vi "SMR_LabVIEW_V1.vi"() -> ()   [LabVIEW 2025]
uses:
  <vilib>/DAQmx/read.llb/DAQmx Read (Analog 1D DBL NChan 1Samp).vi
  <vilib>/Analysis/baseanly.llb/Mean (DBL).vi
  <vilib>/DAQmx/create/channels.llb/DAQmx Create Channel (AI-Temperature-Thermocouple).vi
  <vilib>/DAQmx/create/channels.llb/DAQmx Create Channel (AI-Voltage-Basic).vi
  <vilib>/DAQmx/miscellaneous.llb/DAQmx Fill In Error Info.vi
  <vilib>/Analysis/NI_AALBase.lvlib
panel:
  out "Temperatures T1-T8 (deg C)":dbl[](array[numeric])
  out "Flow History":dbl(graph)
  out "Pressure History":dbl[](graph)
  out "Temperature History":dbl[](graph)
  out "Max Loop Pressure (psi)":dbl
  out "Average Loop Temp (deg C)":dbl
  out "Max Loop Temp (deg C)":dbl
  out "Heat Exchanger Flow (GPM)":dbl
  out "Raw NI9201 Voltages (V)":dbl[](array[numeric])
  out "Pressures P1-P7 (psi)":dbl[](array[numeric])
  in  "Loop Period (ms)":dbl=1000.0
  in  "Stop":bool
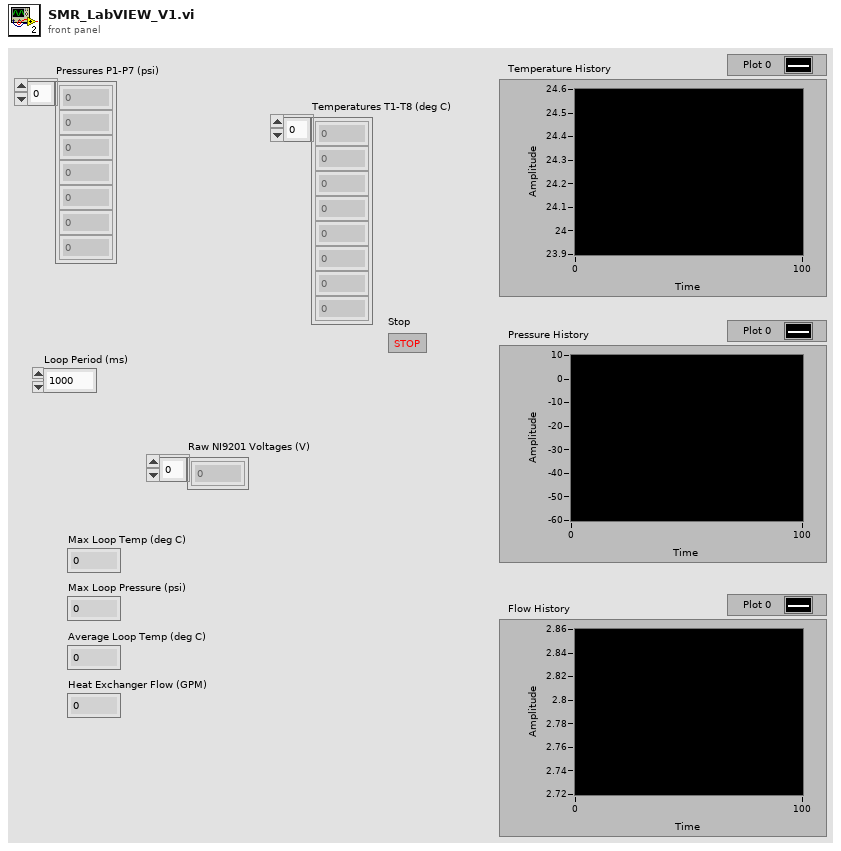
[diagram p1: front panel]
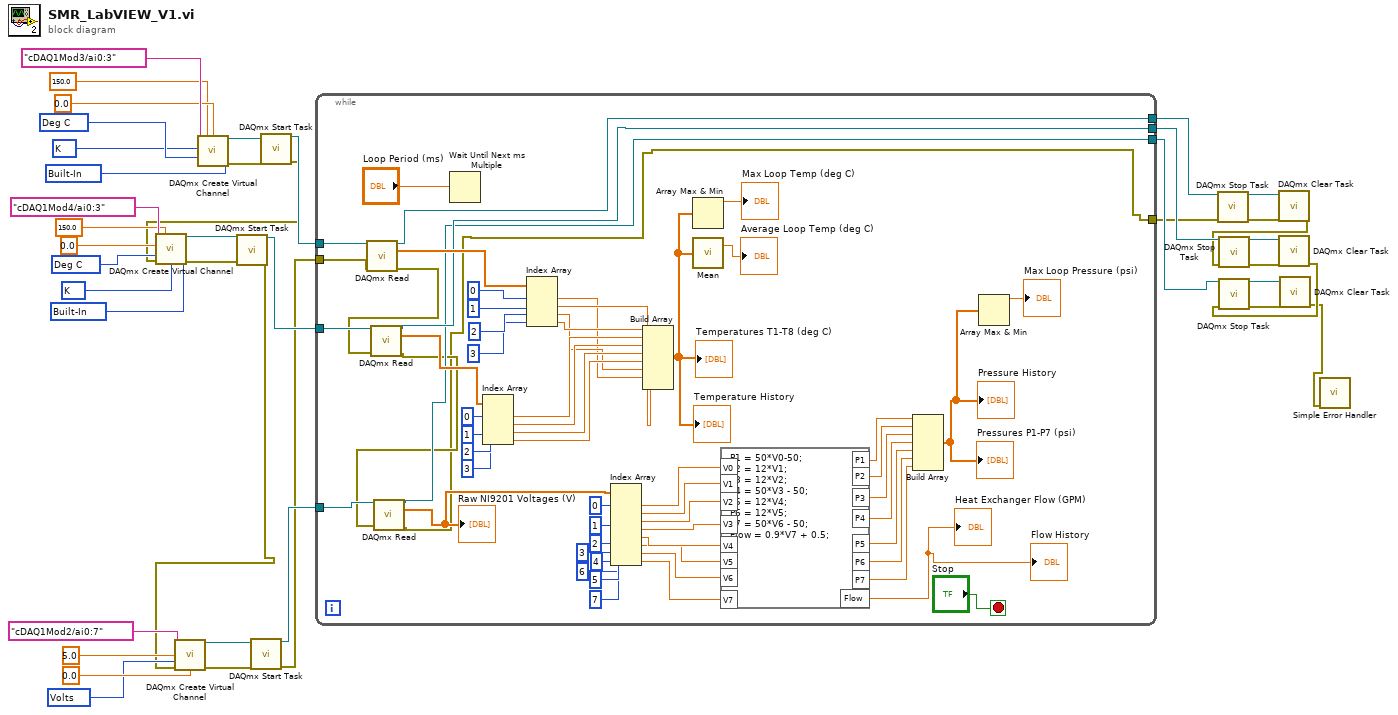
[diagram p0: block diagram]
diagram:
  w23 = 10348 items=["Volts"=10348, "From Custom Scale"=10065] ("units")
  w27 = 10200 items=["Built-In"=10200, "Constant Value"=10116, "Channel"=10113] ("cjc source")
  w28 = 10073 items=["J"=10072, "K"=10073, "N"=10077, "R"=10082, "S"=10085, "T"=10086, "B"=10047, "E"=10055] ("thermocouple type")
  w11 = 10143 items=["Deg C"=10143, "Deg F"=10144, "Kelvins"=10325, "Deg R"=10145, "From Custom Scale"=10065] ("units")
  w31 = 10200 items=["Built-In"=10200, "Constant Value"=10116, "Channel"=10113] ("cjc source")
  w32 = 10073 items=["J"=10072, "K"=10073, "N"=10077, "R"=10082, "S"=10085, "T"=10086, "B"=10047, "E"=10055] ("thermocouple type")
  w35 = 10143 items=["Deg C"=10143, "Deg F"=10144, "Kelvins"=10325, "Deg R"=10145, "From Custom Scale"=10065] ("units")
  n1 = call-poly <vilib>:"DAQmx Create Virtual Channel.vi"("maximum value"=150.0, "minimum value"=0.0, "physical channels"=tag "cDAQ1Mod3/ai0:3", "cjc source"=w31, "units"=w35, "thermocouple type"=w32) -> ("task out"=w40:refnum<k21>, "error out"=w39:errorcluster)  [unwired: 8 in]
  n2 = call <vilib>:"DAQmx Start Task.vi"("task/channels in"=w40, "error in"=w39) -> ("task out"=w20:refnum<k21>, "error out"=w10:errorcluster)  [unwired: 12 in]
  n3 = call-poly <vilib>:"DAQmx Create Virtual Channel.vi"("maximum value"=150.0, "minimum value"=0.0, "physical channels"=tag "cDAQ1Mod4/ai0:3", "cjc source"=w27, "units"=w11, "error in"=w10, "thermocouple type"=w28) -> ("task out"=w37:refnum<k21>, "error out"=w36:errorcluster)  [unwired: 7 in]
  n4 = call <vilib>:"DAQmx Start Task.vi"("task/channels in"=w37, "error in"=w36) -> ("task out"=w19:refnum<k21>, "error out"=w9:errorcluster)  [unwired: 12 in]
  n5 = call-poly <vilib>:"DAQmx Create Virtual Channel.vi"("maximum value"=5.0, "minimum value"=0.0, "physical channels"=tag "cDAQ1Mod2/ai0:7", "units"=w23, "error in"=w9) -> ("task out"=w22:refnum<k21>, "error out"=w21:errorcluster)  [unwired: 9 in]
  n6 = call <vilib>:"DAQmx Start Task.vi"("task/channels in"=w22, "error in"=w21) -> ("task out"=w18:refnum<k21>, "error out"=w8:errorcluster)  [unwired: 12 in]
  n7 = while {
    tunnel: w20 -> [w99]
    tunnel: w19 -> [w98]
    tunnel: w18 -> [w76]
    tunnel: [w48] -> w17
    tunnel: [w47] -> w16
    tunnel: [w46] -> w15
    tunnel: w8 -> [w45]
    tunnel: [w42] -> w7
    stop <- "Stop" stop-if-true
    n8 = call-poly <vilib>:"DAQmx Read.vi"("task/channels in"=w99, "error in"=w45) -> ("task out"=w48:refnum<k21>, "data"=w81:dbl[], "error out"=w44:errorcluster)  [unwired: 11 in]
    n9 = call-poly <vilib>:"DAQmx Read.vi"("task/channels in"=w98, "error in"=w44) -> ("task out"=w47:refnum<k21>, "data"=w80:dbl[], "error out"=w43:errorcluster)  [unwired: 11 in]
    n10 = call-poly <vilib>:"DAQmx Read.vi"("task/channels in"=w76, "error in"=w43) -> ("task out"=w46:refnum<k21>, "data"=w67:dbl[], "error out"=w42:errorcluster)  [unwired: 11 in]
    "Raw NI9201 Voltages (V)" <- w67
    n11 = Wait Until Next ms Multiple(millisecond multiple="Loop Period (ms)") -> ()  [unwired: 1 out]
    n12 = Index Array(array=w80, index #1=0 ("index"), index #2=1 ("index"), index #3=2 ("index"), index #4=3 ("index")) -> (element #1=w89:dbl, element #2=w88:dbl, element #3=w87:dbl, element #4=w86:dbl)
    n13 = Index Array(array=w81, index #1=0 ("index"), index #2=1 ("index"), index #3=2 ("index"), index #4=3 ("index")) -> (element #1=w82:dbl, element #2=w83:dbl, element #3=w84:dbl, element #4=w85:dbl)
    n14 = Index Array(array=w67, index #1=0 ("index"), index #2=1 ("index"), index #3=2 ("index"), index #4=3 ("index"), index #5=4 ("index"), index #6=5 ("index"), index #7=6 ("index"), index #8=7 ("index")) -> (element #1=w66:dbl, element #2=w65:dbl, element #3=w64:dbl, element #4=w63:dbl, element #5=w62:dbl, element #6=w61:dbl, element #7=w60:dbl, element #8=w59:dbl)
    n15 = Build Array(w85, w89, w88, w87, w86, w84, w82, w83) -> (w78:dbl[])
    "Temperatures T1-T8 (deg C)" <- w78
    "Temperature History" <- w78
    n16 = Array Max & Min(array=w78) -> (max value=→"Max Loop Temp (deg C)":dbl)  [unwired: 3 out]
    n17 = call-poly <vilib>:"Mean.vi"("X"=w78) -> ("mean"=→"Average Loop Temp (deg C)":dbl)  [unwired: 1 out]
    n18 = formula code="P1 = 50*V0-50;\nP2 = 12*V1;\nP3 = 12*V2;\nP4 = 50*V3 - 50;\nP5 = 12*V4;\nP6 = 12*V5; \nP7 = 50*V6 - 50;\nFlow = 0.9*V7 + 0.5;"("V0"=w66, "V1"=w65, "V2"=w64, "V3"=w63, "V4"=w62, "V5"=w61, "V6"=w60, "V7"=w59) -> ("P1"=w58:dbl, "P2"=w57:dbl, "P3"=w56:dbl, "P4"=w55:dbl, "P5"=w54:dbl, "P6"=w53:dbl, "P7"=w52:dbl, "Flow"=→"Heat Exchanger Flow (GPM)" →"Flow History":dbl)
    n19 = Build Array(w58, w57, w56, w55, w54, w53, w52) -> (w51:dbl[])
    "Pressures P1-P7 (psi)" <- w51
    "Pressure History" <- w51
    n20 = Array Max & Min(array=w51) -> (max value=→"Max Loop Pressure (psi)":dbl)  [unwired: 3 out]
  }
  n21 = call <vilib>:"DAQmx Stop Task.vi"("task/channels in"=w17, "error in"=w7) -> ("task out"=w14:refnum<k21>, "error out"=w6:errorcluster)  [unwired: 12 in]
  n22 = call <vilib>:"DAQmx Clear Task.vi"("task in"=w14, "error in"=w6) -> ("error out"=w5:errorcluster)  [unwired: 13 in]
  n23 = call <vilib>:"DAQmx Stop Task.vi"("task/channels in"=w16, "error in"=w5) -> ("task out"=w13:refnum<k21>, "error out"=w4:errorcluster)  [unwired: 12 in]
  n24 = call <vilib>:"DAQmx Clear Task.vi"("task in"=w13, "error in"=w4) -> ("error out"=w3:errorcluster)  [unwired: 13 in]
  n25 = call <vilib>:"DAQmx Stop Task.vi"("task/channels in"=w15, "error in"=w3) -> ("task out"=w12:refnum<k21>, "error out"=w2:errorcluster)  [unwired: 12 in]
  n26 = call <vilib>:"DAQmx Clear Task.vi"("task in"=w12, "error in"=w2) -> ("error out"=w1:errorcluster)  [unwired: 13 in]
  n27 = call <vilib>:"Simple Error Handler.vi"("error in (no error)"=w1) -> ()  [unwired: 4 in, 5 out]
